vi "read torque.vi"(8 "error in (no error)":errorcluster, 11 "Torque Transducer in":refnum<class "Torque Transducer.lvclass">) -> (0 "error out":errorcluster, 3 "Torque Transducer out":refnum<class "Torque Transducer.lvclass">)   [LabVIEW 2025, in "Torque Transducer.lvclass"]
uses:
  Torque Transducer.lvclass
  Torque Transducer.lvclass/Torque Transducer.ctl
  <vilib>/DAQmx/read.llb/DAQmx Read (Analog DBL 1Chan 1Samp).vi
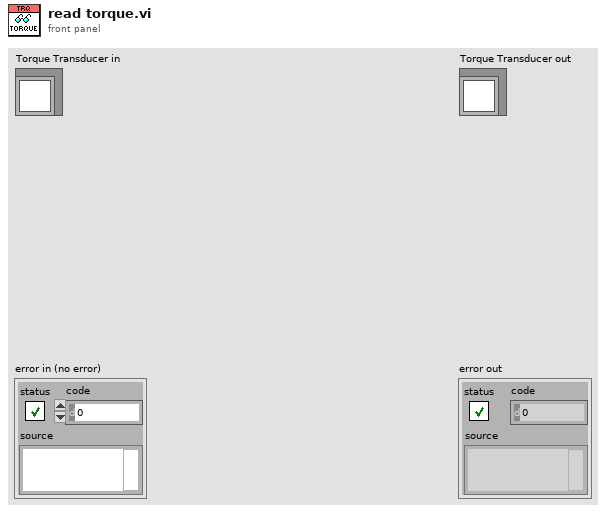
[diagram p1: front panel]
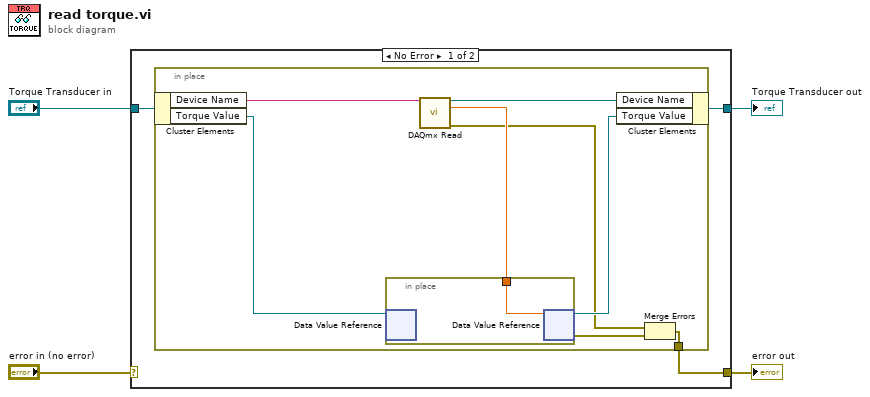
[diagram p0: block diagram]
diagram:
  n1 = case shown="No Error" "error in (no error)" {
    selector: "error in (no error)" -> [_ w18]
    tunnel: [w6 w18] -> w3
    tunnel: [w5 w17] -> w1
    tunnel: "Torque Transducer in" -> [w7 w17]
    frame No Error {
      n2 = in-place {
        in-place-border: [w8] -> w6
        n3 = in-place-cluster #1(w7) -> ("Device Name"=w13:string, "Torque Value"=w15:refnum<data-value>)
        n4 = call-poly <vilib>:"DAQmx Read.vi"("task/channels in"=w13) -> ("task out"=w11:refnum<k21>, "data"=w12:dbl, "error out"=w9:errorcluster)  [unwired: 12 in]
        n5 = in-place {
          in-place-border: w12 -> [w16]
          n6 = in-place-dvr #2(w15) -> ()  [unwired: 2 out]
          n7 = in-place-dvr #2(w16) -> (w14:refnum<data-value>, w10:errorcluster)
        }
        n8 = in-place-cluster #1("Device Name"=w11, "Torque Value"=w14) -> (w5:refnum<class "Torque Transducer.lvclass">)
        n9 = Merge Errors(w9, w10) -> (w8:errorcluster)
      }
    }
    frame Error {
    }
  }
  "error out" <- w3
  "Torque Transducer out" <- w1
